vi "36.vi"() -> ()   [LabVIEW 2021]
panel:
  out "sum":u64
  in  "N_max":i32
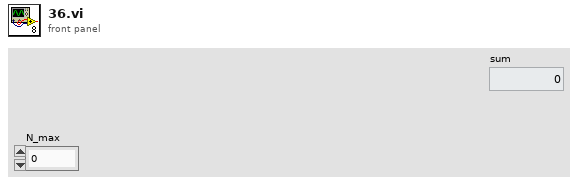
[diagram p1: front panel]
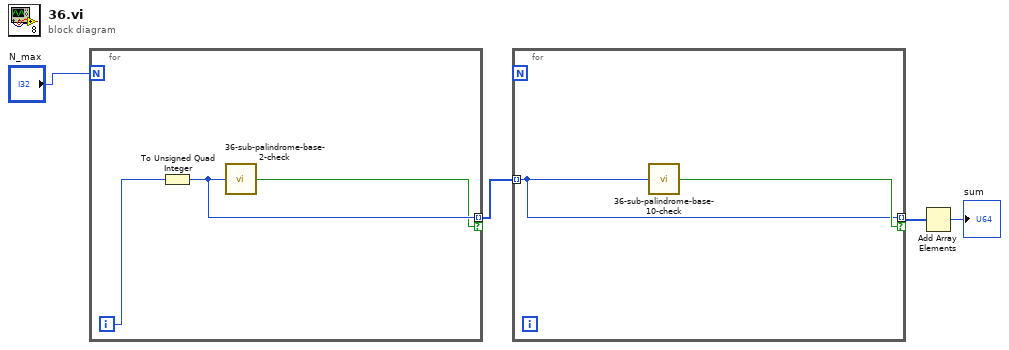
[diagram p0: block diagram]
diagram:
  n1 = for {
    N: "N_max" -> [_]
    tunnel: [w6] -> w3 mode=indexing if=w5
    i -> [w7]
    n2 = To Unsigned Quad Integer(1:w7) -> (0:w6:u64)
    n3 = call "36-sub-palindrome-base-2-check.vi"("Number"=w6) -> ("Number is Palindrome in Base 2?"=w5:bool)
  }
  n4 = for {
    tunnel: [w8] -> w2 mode=indexing if=w9
    tunnel: w3 -> [w8] mode=indexing
    n5 = call "36-sub-palindrome-base-10-check.vi"("Number"=w8) -> ("Number is Palindrome in Base 10?"=w9:bool)
  }
  n6 = Add Array Elements(numeric array=w2) -> (sum=→"sum":u64)
